vi "createGroup.vi"(8 "error in (no error)":errorcluster, 10 "Velocity":dbl=0.1, 11 "VISA Refnum in":refnum<visa-resource-name>) -> (0 "error out":errorcluster, 3 "VISA Refnum out":refnum<visa-resource-name>)   [LabVIEW 2014]
doc: "Newport Motion Controler\nThis VI create a Group\n\nAndré Romero - 2022\nandretec@ifsc.usp.br"
uses:
  <userlib>/Newport ESP301/Newport ESP301.lvlib
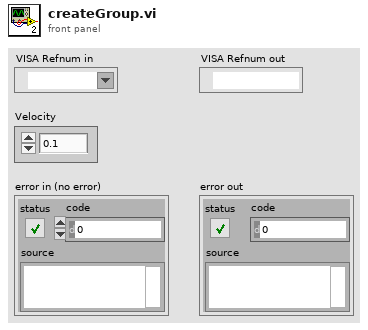
[diagram p1: front panel]
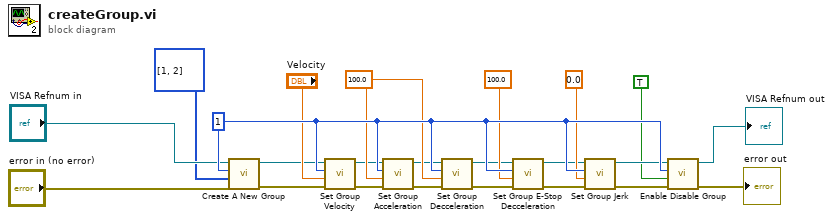
[diagram p0: block diagram]
diagram:
  w23 = 1 ("Group #")
  w9 = 100.0 ("Acceleration (0 units/s²)")
  n1 = call <userlib>:"Create A New Group.vi"("error in (no error)"="error in (no error)", "Axis Number"=i32[] [1, 2], "Group Number (1)"=w23, "VISA resource name"="VISA Refnum in") -> ("error out"=w3:errorcluster, "VISA resource name out"=w2:refnum<visa-resource-name>)  [unwired: 2 in]
  n2 = call <userlib>:"Set Group Velocity.vi"("error in (no error)"=w3, "Velocity (units/s)"="Velocity", "Group Number (1)"=w23, "VISA resource name"=w2) -> ("error out"=w8:errorcluster, "VISA resource name out"=w5:refnum<visa-resource-name>)  [unwired: 2 in]
  n3 = call <userlib>:"Set Group Acceleration.vi"("error in (no error)"=w8, "Acceleration (0 units/s²)"=w9, "Group Number (1)"=w23, "VISA resource name"=w5) -> ("error out"=w7:errorcluster, "VISA resource name out"=w6:refnum<visa-resource-name>)  [unwired: 2 in]
  n4 = call <userlib>:"Set Group Decceleration.vi"("error in (no error)"=w7, "Decceleration (0 units/s²)"=w9, "Group Number (1)"=w23, "VISA resource name"=w6) -> ("error out"=w13:errorcluster, "VISA resource name out"=w10:refnum<visa-resource-name>)  [unwired: 2 in]
  n5 = call <userlib>:"Set Group E-Stop Decceleration.vi"("error in (no error)"=w13, "E-Stop Decceleration (0 units/s²)"=100.0, "Group Number (1)"=w23, "VISA resource name"=w10) -> ("error out"=w14:errorcluster, "VISA resource name out"=w11:refnum<visa-resource-name>)  [unwired: 2 in]
  n6 = call <userlib>:"Set Group Jerk.vi"("error in (no error)"=w14, "Vector Jerk (0 units/s^3)"=0.0, "Group Number (1)"=w23, "VISA resource name"=w11) -> ("error out"=w15:errorcluster, "VISA resource name out"=w12:refnum<visa-resource-name>)  [unwired: 2 in]
  n7 = call <userlib>:"Enable Disable Group.vi"("error in (no error)"=w15, "Action (OFF)"=TRUE, "Group Number (1)"=w23, "VISA resource name"=w12) -> ("error out"=→"error out":errorcluster, "VISA resource name out"=→"VISA Refnum out":refnum<visa-resource-name>)  [unwired: 2 in]
